vi "Ventilator Control.vi"(2 "error in (no error)":errorcluster, 3 "Ventilator (off)":bool, 4 "Lines read":tag, 5 "Lines write":tag) -> (0 "error out":errorcluster, 1 "Ventilator State":bool)   [LabVIEW 2021]
doc: "Controla la activación y desactivación del ventilador de una DAQ"
uses:
  <vilib>/DAQmx/write.llb/DAQmx Write (Digital Bool 1Line 1Point).vi
  <vilib>/DAQmx/read.llb/DAQmx Read (Digital Bool 1Line 1Point).vi
  <vilib>/DAQmx/create/channels.llb/DAQmx Create Channel (DO-Digital Output).vi
  <vilib>/DAQmx/miscellaneous.llb/DAQmx Fill In Error Info.vi
  <vilib>/DAQmx/create/channels.llb/DAQmx Create Channel (DI-Digital Input).vi
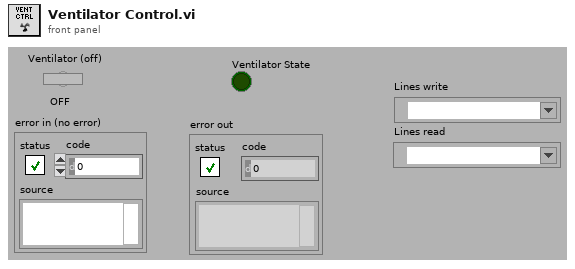
[diagram p1: front panel]
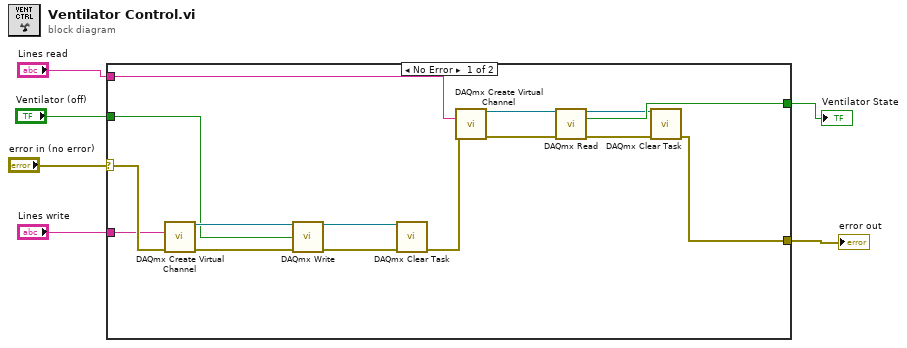
[diagram p0: block diagram]
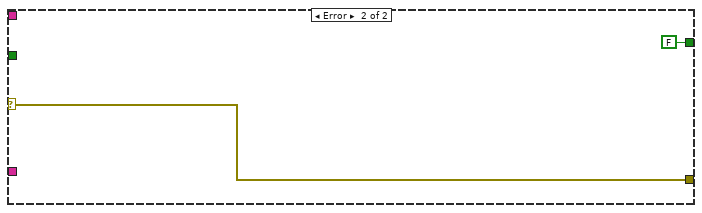
[diagram p2: hidden frame]
diagram:
  n1 = case shown="No Error" "error in (no error)" {
    selector: "error in (no error)" -> [w21 w23]
    tunnel: [w12 w23] -> w5
    tunnel: "Ventilator (off)" -> [w16 _]
    tunnel: [w11 FALSE ("data")] -> w3
    tunnel: "Lines write" -> [w8 _]
    tunnel: "Lines read" -> [w7 _]
    frame No Error {
      n2 = call-poly <vilib>:"DAQmx Create Virtual Channel.vi"("lines"=w8, "error in"=w21) -> ("task out"=w18:refnum<k21>, "error out"=w20:errorcluster)  [unwired: 12 in]
      n3 = call-poly <vilib>:"DAQmx Write.vi"("task/channels in"=w18, "data"=w16, "error in"=w20) -> ("task out"=w17:refnum<k21>, "error out"=w19:errorcluster)  [unwired: 10 in, 1 out]
      n4 = call <vilib>:"DAQmx Clear Task.vi"("task in"=w17, "error in"=w19) -> ("error out"=w15:errorcluster)  [unwired: 13 in]
      n5 = call-poly <vilib>:"DAQmx Create Virtual Channel.vi"("lines"=w7, "error in"=w15) -> ("task out"=w10:refnum<k21>, "error out"=w14:errorcluster)  [unwired: 12 in]
      n6 = call-poly <vilib>:"DAQmx Read.vi"("task/channels in"=w10, "error in"=w14) -> ("task out"=w9:refnum<k21>, "data"=w11:bool, "error out"=w13:errorcluster)  [unwired: 11 in]
      n7 = call <vilib>:"DAQmx Clear Task.vi"("task in"=w9, "error in"=w13) -> ("error out"=w12:errorcluster)  [unwired: 13 in]
    }
    frame Error {
    }
  }
  "error out" <- w5
  "Ventilator State" <- w3
